vi "Start Active DUT Power Cycle.vi"(8 "error in (no error)":errorcluster, 11 "VISA resource name":refnum<visa-resource-name>) -> (0 "error out":errorcluster, 3 "VISA resource name out":refnum<visa-resource-name>)   [LabVIEW 2020, in "Rohde&Schwarz CMXP Base.lvlib"]
doc: "Starts a power cycle at the DUT.\n\nAttribute:\nRSCMXPBASE_ATTR_ACTIVE_DUT_POWER_CYCLE_START\n\nRemote-control command:\nPROCedure:DUT:CONTrol:PCYCle"
uses:
  <instrlib>/Rohde&Schwarz CMXP Base/Rohde&Schwarz CMXP Base.lvlib
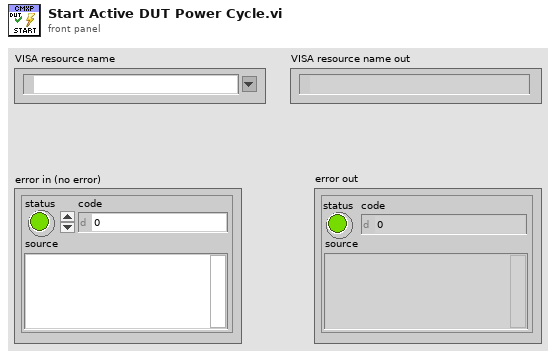
[diagram p1: front panel]
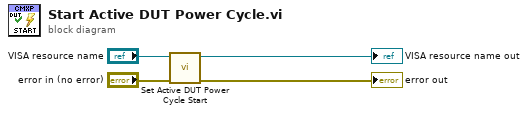
[diagram p0: block diagram]
diagram:
  n1 = call "Set Active DUT Power Cycle Start"("error in (no error)"="error in (no error)", "instrument handle"="VISA resource name") -> ("error out"=→"error out":errorcluster, "instrument handle out"=→"VISA resource name out":refnum<visa-resource-name>)  [unwired: 8 in]
